vi "PhidgetGetIsRemote.vi"(0 "error in (no error)":errorcluster, 3 "Device In":u64) -> (7 "error out":errorcluster, 9 "Remote":bool, 10 "Device Out":u64)   [LabVIEW 2012, in "Phidget Common.lvlib"]
doc: "${IsRemote:Header}"
uses:
  <instrlib>/Phidgets/Phidget Common/Phidget Common.lvlib
  phidget22.dll
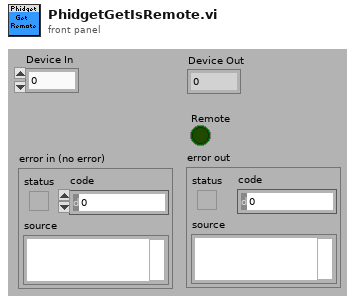
[diagram p1: front panel]
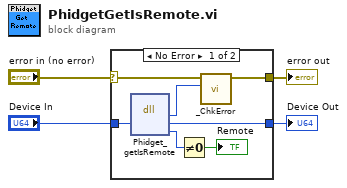
[diagram p0: block diagram]
diagram:
  n1 = case shown="No Error" "error in (no error)" {
    selector: "error in (no error)" -> [w11 w13]
    tunnel: [w10 w13] -> w3
    tunnel: "Device In" -> [w8 w12]
    tunnel: [w9 w12] -> w1
    frame No Error {
      n2 = dll-call lib="phidget22.dll" fn="Phidget_getIsRemote"("phid"=w8) -> ("return type"=w7:i32, "phid"=w9:u64, "Channel"=w6:i32)  [unwired: 4 in, 2 out]
      n3 = Not Equal To 0?(x=w6) -> (x != 0?=→"Remote":bool)
      n4 = call <instrlib>:"_ChkError.vi"("Return Code"=w7, "error in (no error)"=w11) -> ("error out"=w10:errorcluster)  [unwired: 9 in]
    }
    frame Error {
    }
  }
  "error out" <- w3
  "Device Out" <- w1
